vi "Check for Image List.vi"(8 "error in":errorcluster, 11 "TSC Button Editor in":refnum<class "TSC Button Editor.lvclass">) -> (0 "error out":errorcluster, 3 "TSC Button Editor out":refnum<class "TSC Button Editor.lvclass">, 4 "Images":T1(array[cluster]))   [LabVIEW 2021, in "TSC Button Editor.lvclass"]
doc: "This VI will look to see if an image directory binary file exists.\n\n<b>Code Developed By:</b>\nTechnology Service Corporation\nwww.tsc.com/atcs\n\nDeveloper:\nDaniel Coons"
uses:
  TSC Button Editor.lvclass
  TSC Button Editor.lvclass/TSC Button Editor.ctl
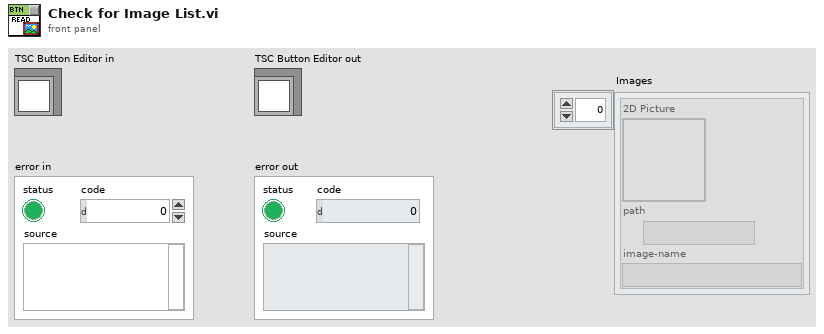
[diagram p1: front panel]
types:
  T1 = cluster{"2D Picture":picture, "path":path, "image-name":string}[]
  T2 = enum16{"open", "replace", "create", "open or create", "replace or create", "replace or create with confirmation"}
  T3 = cluster{"2D Picture":picture, "path":path, "image-name":string}
  T4 = typedef "imagedata.ctl" = cluster{"image type":i32, "image depth":i32, "image":u8[], "mask":u8[], "colors":u32[], "Rectangle":cluster{"left":i16, "top":i16, "right":i16, "bottom":i16}}
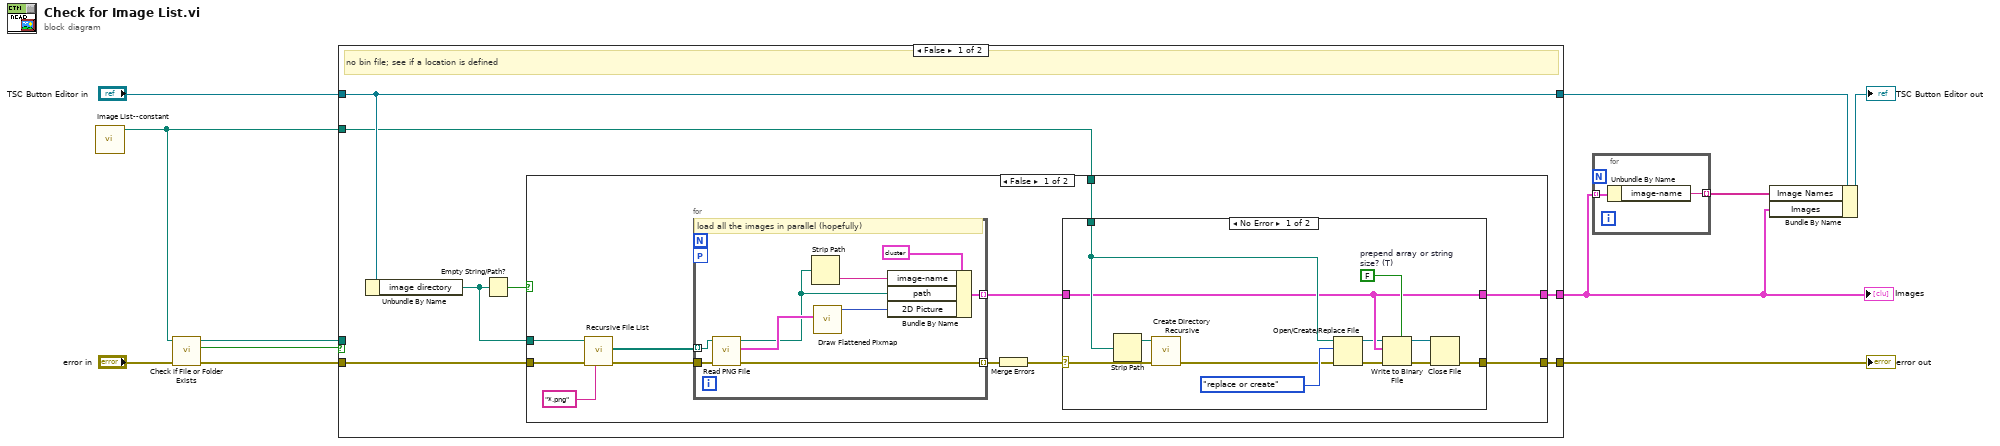
[diagram p0: block diagram]
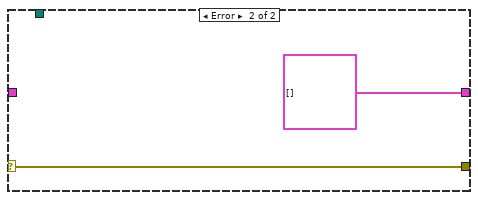
[diagram p2: hidden frame]
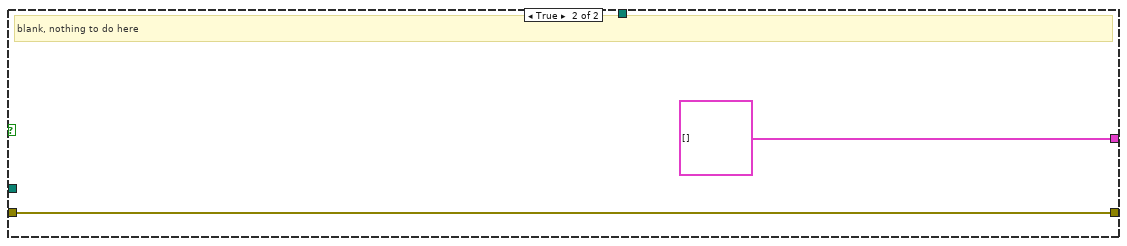
[diagram p3: hidden frame]
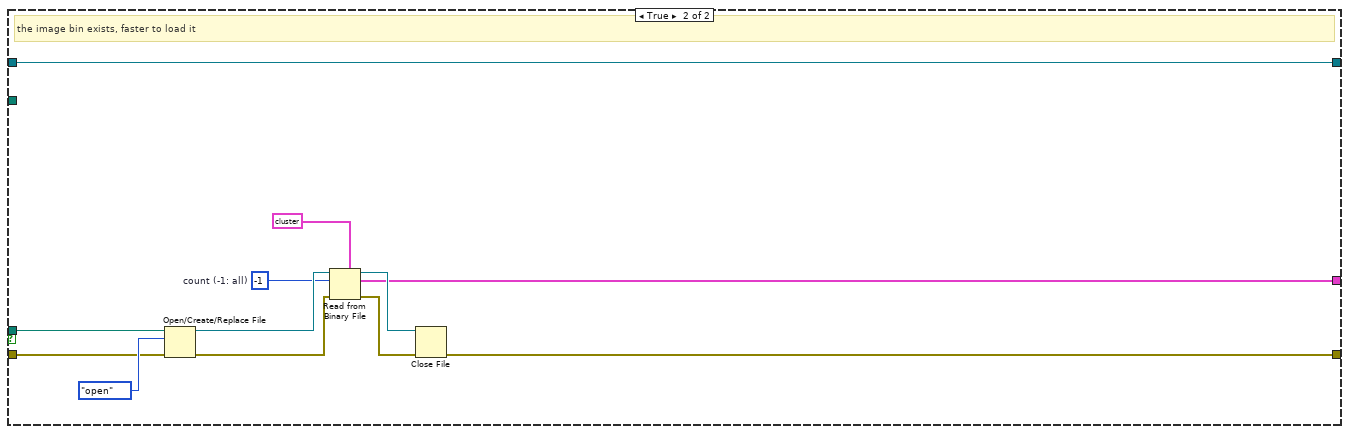
[diagram p4: hidden frame]
diagram:
  n1 = call "Image List--constant.vi"() -> ("image-list"=w2:path)  [unwired: 11 in]
  n2 = call <vilib>:"Check if File or Folder Exists.vi"("error in (no error)"="error in", "path"=w2) -> ("error out"=w9:errorcluster, "file or folder exists?"=w7:bool, "dup path"=w10:path)  [unwired: 7 in]
  n3 = case shown="False" w7 {
    tunnel: w10 -> [_ w59]
    tunnel: w9 -> [w17 w58]
    tunnel: [w16 w57] -> w8
    tunnel: [w18 w56] -> w5
    tunnel: "TSC Button Editor in" -> [w18 w56]
    tunnel: [w13 w55] -> w1
    tunnel: w2 -> [w12 _]
    frame False {
      # "no bin file; see if a location is defined"
      n4 = Unbundle By Name(w18) -> ("image directory"=w14:path)
      n5 = Empty String/Path?(string/path=w14) -> (empty?=w15:bool)
      n6 = case shown="False" w15 {
        tunnel: w17 -> [w28 w54]
        tunnel: [w23 w54] -> w16
        tunnel: w14 -> [w27 _]
        tunnel: [w20 T1 []] -> w13
        tunnel: w12 -> [w19 _]
        frame False {
          n7 = call <vilib>:"Recursive File List.vi"("pattern"="*.png", "error in (no error)"=w28, "Folder Path"=w27) -> ("error out"=w26:errorcluster, "All Files in Dir"=w25:path[])  [unwired: 4 in, 3 out]
          n8 = for {
            tunnel: w25 -> [w52] mode=indexing
            tunnel: [w50] -> w21 mode=indexing
            workers-P: _ -> [_]
            tunnel: w26 -> [w45]
            tunnel: [w44] -> w24 mode=indexing
            # "load all the images in parallel (hopefully)"
            n9 = call <vilib>:"Read PNG File.vi"("error in (no error)"=w45, "path to PNG file"=w52) -> ("error out"=w44:errorcluster, "image data"=w51:T4, "path"=w47:path)  [unwired: 7 in]
            n10 = Strip Path(path=w47) -> (name=w46:string)  [unwired: 1 out]
            n11 = call <vilib>:"Draw Flattened Pixmap.vi"("image data"=w51) -> ("new picture"=w48:picture)  [unwired: 8 in]
            n12 = Bundle By Name(cluster=T3 {"2D Picture"=bytes[0], "path"=path "", "image-name"=""} ("Cluster"), "image-name"=w46, "path"=w47, "2D Picture"=w48) -> (w50:T3)
          }
          n13 = Merge Errors(w24) -> (w22:errorcluster)
          n14 = case shown="No Error" w22 {
            selector: w22 -> [w39 w43]
            tunnel: [w32 w43] -> w23
            tunnel: w21 -> [w33 _]
            tunnel: [w33 T1 []] -> w20
            tunnel: w19 -> [w36 _]
            frame No Error {
              w34 = FALSE  # prepend array or string size? (T)
              n15 = Strip Path(path=w36) -> (stripped path=w37:path)  [unwired: 1 out]
              n16 = call <vilib>:"Create Directory Recursive.vi"("error in (no error)"=w39, "directory"=w37) -> ("error out"=w38:errorcluster)  [unwired: 3 in, 2 out]
              n17 = Open/Create/Replace File(file path (use dialog)=w36, error in=w38, operation (0:open)=T2."replace or create") -> (refnum out=w31:refnum<file>, error out=w41:errorcluster)  [unwired: 3 in, 1 out]
              n18 = Write to Binary File(file (use dialog)=w31, data=w33, error in=w41, 5:w34) -> (refnum out=w30:refnum<file>, error out=w35:errorcluster)  [unwired: 2 in, 1 out]
              n19 = Close File(refnum=w30, error in=w35) -> (error out=w32:errorcluster)  [unwired: 1 out]
            }
            frame Error {
            }
          }
        }
        frame True {
          # "blank, nothing to do here"
        }
      }
    }
    frame True {
      w63 = -1  # count (-1: all)
      # "the image bin exists, faster to load it"
      n20 = Open/Create/Replace File(file path (use dialog)=w59, error in=w58, operation (0:open)=T2."open") -> (refnum out=w64:refnum<file>, error out=w65:errorcluster)  [unwired: 3 in, 1 out]
      n21 = Read from Binary File(5:T3 {"2D Picture"=bytes[0], "path"=path "", "image-name"=""} ("Cluster"), 8:w65, 10:w63, 11:w64) -> (0:w62:errorcluster, 2:w55:T1, 3:w61:refnum<file>)  [unwired: 2 in, 1 out]
      n22 = Close File(refnum=w61, error in=w62) -> (error out=w57:errorcluster)  [unwired: 1 out]
    }
  }
  "error out" <- w8
  "Images" <- w1
  n23 = for {
    tunnel: w1 -> [w68] mode=indexing
    tunnel: [w67] -> w3 mode=indexing
    n24 = Unbundle By Name(w68) -> ("image-name"=w67:string)
  }
  n25 = Bundle By Name(cluster=w5, "Image Names"=w3, "Images"=w1) -> (→"TSC Button Editor out":refnum<class "TSC Button Editor.lvclass">)
